vi "Insert String DB (SubVI).vi"(0 "String Insert":string, 5 "Array":string[](array[string]), 7 "index":i32, 9 "Refnum in":T1, 11 "error in":errorcluster) -> (6 "output array":string[](array[string]), 10 "Refnum in 2":T1, 15 "error out":errorcluster)   [LabVIEW 2012]
uses:
  <vilib>/addons/database/Connection.llb/Conn ObjectReference.ctl
  <vilib>/addons/database/NI_Database_API.lvlib
panel:
  out "x = y?":bool
  out "element":string
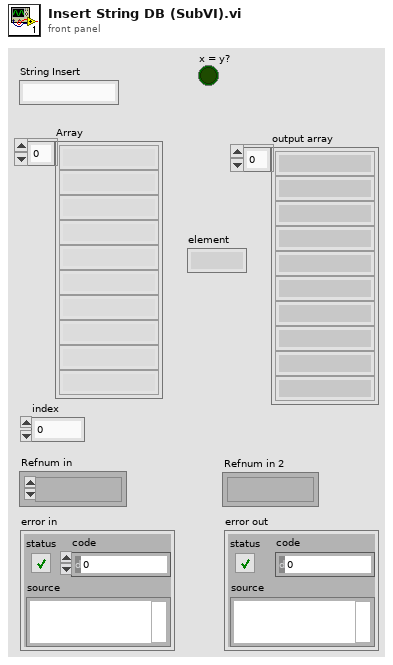
[diagram p1: front panel]
types:
  T1 = typedef "NI_Database_API.lvlib/Conn ObjectReference.ctl" = refnum<k1>
  T2 = cluster{"Imei":string, "Evento":string, "Lat":string, "Lon":string, "F_H_eve":timestamp, "F_H_rec":timestamp}
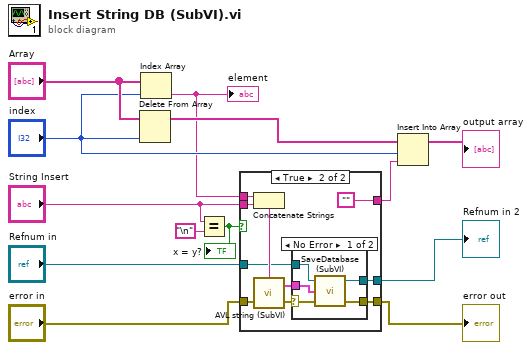
[diagram p0: block diagram]
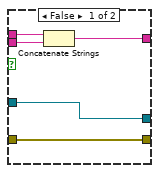
[diagram p2: hidden frame]
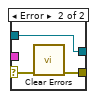
[diagram p3: hidden frame]
diagram:
  n1 = Delete From Array(array="Array", index="index") -> (array with subset deleted=w12:string[])  [unwired: 1 in, 1 out]
  n2 = Index Array(array="Array", index="index") -> (element=w9:string)
  "element" <- w9
  n3 = Equal?(x="String Insert", y="\n") -> (x = y?=w5:bool)
  "x = y?" <- w5
  n4 = case shown="True" w5 {
    tunnel: w9 -> [w18 w28]
    tunnel: [w16 ""] -> w8
    tunnel: "String Insert" -> [w17 w27]
    tunnel: "Refnum in" -> [w15 w22]
    tunnel: "error in" -> [w14 w21]
    tunnel: [w15 w20] -> w2
    tunnel: [w14 w19] -> w1
    frame False {
      n5 = Concatenate Strings(w18, w17) -> (w16:string)
    }
    frame True {
      n6 = Concatenate Strings(w28, w27) -> (w25:string)
      n7 = call "AVL string (SubVI).vi"("error in"=w21, "String"=w25) -> ("error out"=w23:errorcluster, "Datos"=w24:T2)
      n8 = case shown="No Error" w23 {
        selector: w23 -> [w30 w35]
        tunnel: [w33 w36] -> w20
        tunnel: w24 -> [w32 _]
        tunnel: [w31 w34] -> w19
        tunnel: w22 -> [w29 w36]
        frame No Error {
          n9 = call "SaveDatabase (SubVI).vi"("error in (no error)"=w30, "Datos"=w32, "Refnum in"=w29) -> ("error out"=w31:errorcluster, "Refnum out"=w33:T1)  [unwired: 1 in]
        }
        frame Error {
          n10 = call <vilib>:"Clear Errors.vi"("error in (no error)"=w35) -> ("error out"=w34:errorcluster)  [unwired: 6 in]
        }
      }
    }
  }
  "Refnum in 2" <- w2
  "error out" <- w1
  n11 = Insert Into Array(array=w12, index="index", new element=w8) -> (→"output array":string[])
